vi "calculate_servo_PWM.vi"(0 "Angle":dbl, 2 "Servo_gain":dbl, 3 "Servo_bias":dbl) -> (7 "Numeric":u16)   [LabVIEW 2020]
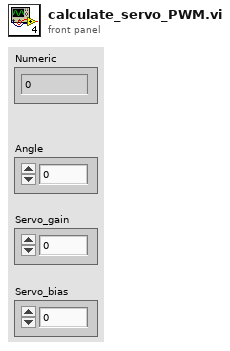
[diagram p1: front panel]
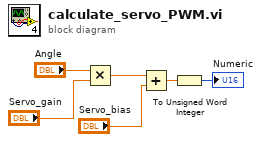
[diagram p0: block diagram]
diagram:
  n1 = Multiply(x="Angle", y="Servo_gain") -> (x*y=w5:dbl)
  n2 = Add(x=w5, y="Servo_bias") -> (x+y=w4:dbl)
  n3 = To Unsigned Word Integer(number=w4) -> (unsigned 16bit integer=→"Numeric":u16)
